vi "mes~产品进站.vi"(8 "error in (no error)":errorcluster caption="错误输入（无错误）", 11 "identification":string caption="identification:") -> (0 "error out":errorcluster caption="错误输出", 1 "ErrorMessage":string, 2 "进站成功":bool)   [LabVIEW 2020]
uses:
  Global.vi
  <vilib>/addons/_JKI.lib/Serialization/JSON/JKI JSON Serialization.lvlib
panel:
  in  "Headers":string[][](array[string])=[["Content-Type", "application/json"]]
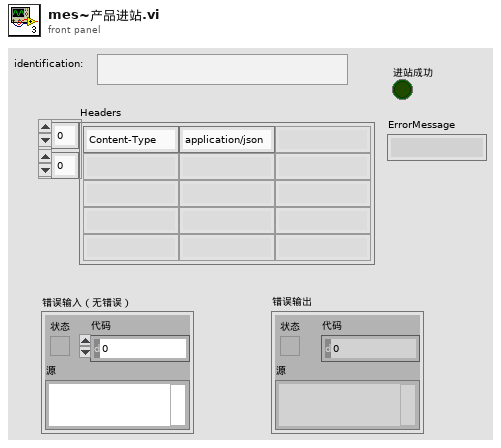
[diagram p1: front panel]
types:
  T1 = cluster{"equipmentCode":string, "productBarcode":string}
  T2 = cluster{"接口地址(URL)":string, "用户登录":string, "产品进站":string, "参数采集":string, "产品出站":string, "设备状态":string, "设备编号(equipNum)":string, "站点名称(siteCode)":string, "生产类型(productType)":string, "追溯编号(traceCode)":string}
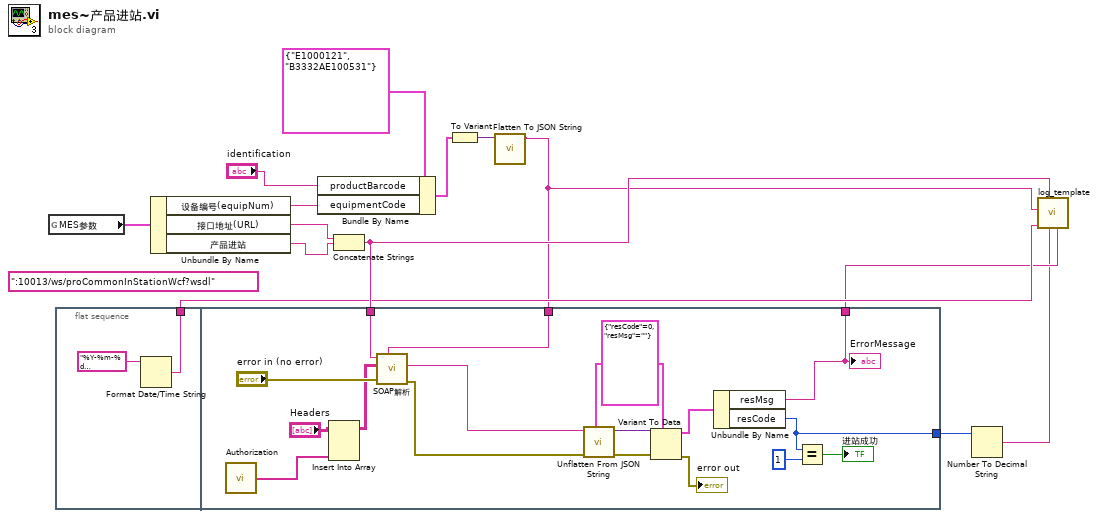
[diagram p0: block diagram]
diagram:
  (unwired) ":10013/ws/proCommonInStationWcf?wsdl"
  n1 = global read "Global.vi" "MES参数"() -> (w12:T2)
  n2 = flat-sequence {
    tunnel: [w15] -> w9
    tunnel: w4 -> [w29]
    tunnel: w10 -> [w30]
    tunnel: [w28] -> w8
    tunnel: [w27] -> w3
    frame #0 {
      n3 = Format Date/Time String(time format string (%c)="%Y-%m-%d %H:%M:%S%3u-->" ("EndTime")) -> (date/time string=w15:string)  [unwired: 2 in]
    }
    frame #1 {
      w26 = cluster{"resCode":i32, "resMsg":string} {"resCode"=0, "resMsg"=""} ("用户登录ctl")
      n4 = call "Authorization.vi"() -> ("Authorization"=w18:string[])
      n5 = Insert Into Array(array="Headers", new element=w18) -> (w17:string[][])  [unwired: 2 in]
      n6 = call "SOAP解析.vi"("DATA"=w29, "错误输入（无错误）"="error in (no error)", "Headers"=w17, "URL"=w30) -> ("错误输出"=w22:errorcluster, "body"=w23:string)  [unwired: 5 in, 1 out]
      n7 = call <vilib>:"Unflatten From JSON String.vi"("Type and Defaults"=w26, "error in (no error)"=w22, "JSON String"=w23) -> ("error out"=w21:errorcluster, "Variant"=w20:variant)  [unwired: 7 in]
      n8 = Variant To Data(error in=w21, type=w26, Variant=w20) -> (data=w33:cluster{"resCode":i32, "resMsg":string}, error out=→"error out":errorcluster)
      n9 = Unbundle By Name(w33) -> ("resMsg"=w28:string, "resCode"=w27:i32)
      "ErrorMessage" <- w28
      n10 = Equal?(x=w27, y=1) -> (x = y?=→"进站成功":bool)
    }
  }
  n11 = Unbundle By Name(w12) -> ("设备编号(equipNum)"=w13:string, "接口地址(URL)"=w1:string, "产品进站"=w11:string)
  n12 = Bundle By Name(cluster=T1 {"equipmentCode"="E1000121", "productBarcode"="B3332AE100531"} ("用户登录ctl"), "productBarcode"="identification", "equipmentCode"=w13) -> (w14:T1)
  n13 = Concatenate Strings(w1, w11) -> (w10:string)
  n14 = To Variant(anything=w14) -> (Variant=w5:variant)
  n15 = call <vilib>:"Flatten To JSON String.vi"("Variant"=w5) -> ("JSON String"=w4:string)  [unwired: 9 in, 1 out]
  n16 = Number To Decimal String(number=w3) -> (decimal integer string=w2:string)  [unwired: 1 in]
  n17 = call "log_template.vi"("接收报文"=w8, "a:Success"=w2, "URL"=w10, "StartTime"=w9, "发送报文"=w4) -> ()  [unwired: 7 in]
